vi "PWM RT1.vi"(10 "占空比":dbl, 11 "频率":u16) -> (2 "F":u32, 3 "T":u32)   [LabVIEW 2017]
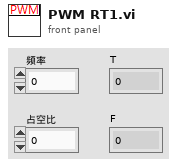
[diagram p1: front panel]
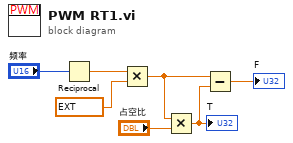
[diagram p0: block diagram]
diagram:
  n1 = Reciprocal ("倒数")(x="频率") -> (1/x=w2:ext)
  n2 = Multiply(x=w2, y=ext 1000000.0) -> (x*y=w4:ext)
  n3 = Multiply(x=w4, y="占空比") -> (x*y=w6:ext)
  "T" <- w6
  n4 = Subtract(x=w4, y=w6) -> (x-y=→"F":ext)
